vi "right shift without data loss.vi"(1 "shift index":i32=2, 2 "x[n]":dbl[](array[numeric])) -> (0 "Right shifted x[n]":dbl[](array[numeric]))   [LabVIEW 2009]
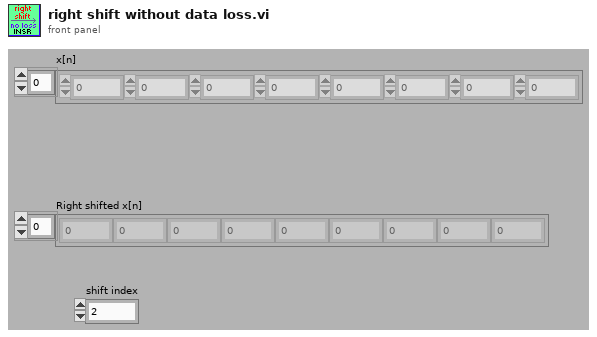
[diagram p1: front panel]
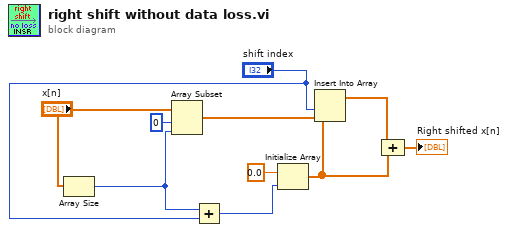
[diagram p0: block diagram]
diagram:
  n1 = Array Size(array="x[n]") -> (size(s)=w3:i32)
  n2 = Array Subset(array="x[n]", index=0, length=w3) -> (w8:dbl[])
  n3 = Add(x=w3, y="shift index") -> (x+y=w1:i32)
  n4 = Initialize Array(0.0 ("element"), w1) -> (w5:dbl[])
  n5 = Insert Into Array(array=w5, index="shift index", new element=w8) -> (w6:dbl[])
  n6 = Compound Arithmetic op=ADD(w6, w5) -> (→"Right shifted x[n]":dbl[])
